vi "NumbertoDVR.vi"(10 "Numeric":i32) -> (2 "FrameworkDataRef":T1)   [LabVIEW 2016, in "EmbeddedMainUI.lvclass"]
uses:
  EmbeddedMainUI.lvclass
  Typedefs/FrameworkDataRef.ctl
  FrameworkData.ctl
  <vilib>/Levylab/Embedded SMO UI/EmbeddedSMO.lvclass
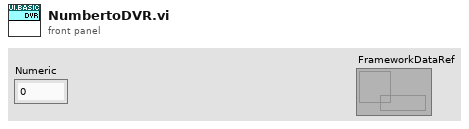
[diagram p1: front panel]
types:
  T1 = typedef "EmbeddedMainUI.lvclass/FrameworkDataRef.ctl" = refnum<data-value>
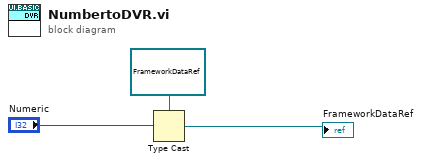
[diagram p0: block diagram]
diagram:
  n1 = Type Cast(type=T1 refnum ("FrameworkDataRef"), x="Numeric") -> (*(type *) &x=→"FrameworkDataRef":T1)
